vi "ExecuteCommand.vi"(10 "Params":string[][](array[string]), 11 "Command":string) -> ()   [LabVIEW 2017]
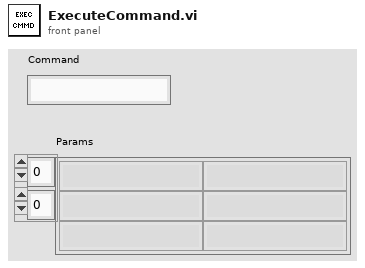
[diagram p1: front panel]
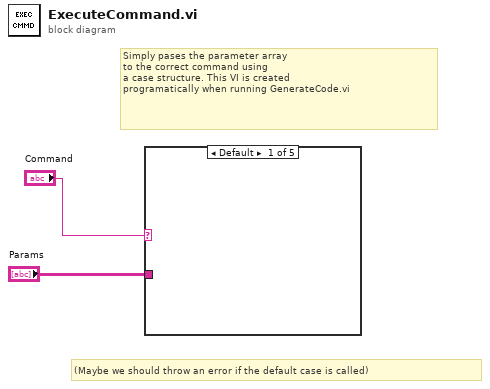
[diagram p0: block diagram]
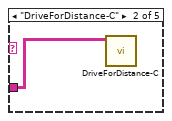
[diagram p2: hidden frame]
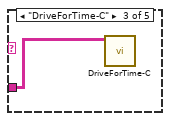
[diagram p3: hidden frame]
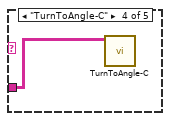
[diagram p4: hidden frame]
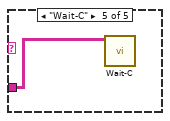
[diagram p5: hidden frame]
diagram:
  # "(Maybe we should throw an error if the default case is called)"
  # "Simply pases the parameter array\nto the correct command using\na case structure. This VI is created\nprogramatically when running GenerateCode.vi"
  n1 = case shown="Default" "Command" {
    tunnel: "Params" -> [_ w3 w4 w5 w6]
    frame Default {
    }
    frame "DriveForDistance-C" {
      n2 = call "DriveForDistance-C.vi"("Params"=w3) -> ()  [unwired: 11 in]
    }
    frame "DriveForTime-C" {
      n3 = call "DriveForTime-C.vi"("Params"=w4) -> ()  [unwired: 11 in]
    }
    frame "TurnToAngle-C" {
      n4 = call "TurnToAngle-C.vi"("Params"=w5) -> ()  [unwired: 11 in]
    }
    frame "Wait-C" {
      n5 = call "Wait-C.vi"("Params"=w6) -> ()  [unwired: 11 in]
    }
  }
